vi "CMD execution.vi"(0 "Command":string="Notepad.exe ", 5 "Path":string, 7 "File name":string, 9 "File type":string, 11 "error in (no error)":errorcluster) -> (15 "error out":errorcluster)   [LabVIEW 2018]
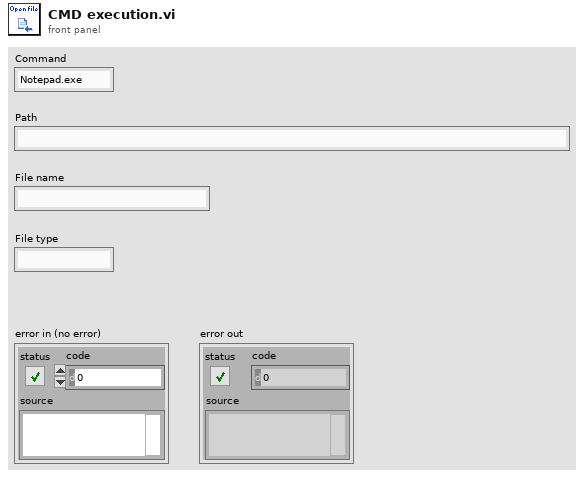
[diagram p1: front panel]
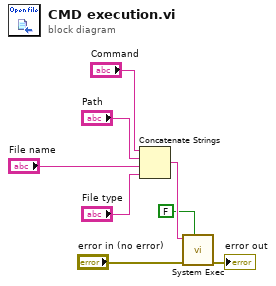
[diagram p0: block diagram]
diagram:
  n1 = Concatenate Strings("Command", "Path", "File name", "File type") -> (w5:string)
  n2 = call <vilib>:"System Exec.vi"("wait until completion? (T)"=FALSE, "error in (no error)"="error in (no error)", "command line"=w5) -> ("error out"=→"error out":errorcluster)  [unwired: 5 in, 3 out]
